vi "Initialize Attributes.vi"(8 "error in (no error)":errorcluster, 10 "Attribute Data":variant, 11 "BNT_DAQmx-MCSV in":refnum<class "BNT_DAQmx-MCSV.lvclass">) -> (0 "error out":errorcluster, 2 "Found?":bool, 3 "BNT_DAQmx-MCSV out":refnum<class "BNT_DAQmx-MCSV.lvclass">)   [LabVIEW 2017, in "BNT_DAQmx.lvlib" / "BNT_DAQmx-MCSV.lvclass"]
doc: "Initialize object attribute.\n\nUnique resources should be allocated elsewhere!"
uses:
  BNT_DAQmx-MCSV.lvclass
  CSPP_Core/Actors/CS++BaseActor/CS++BaseActor.lvclass
  CSPP_Core/Classes/CS++ProcessVariables/ProcessVariable/PV.lvclass
  CSPP_Core/Classes/CS++ProcessVariables/CS++ProcessVariables.lvlib
  CSPP_Core/Actors/CS++DeviceActor/CS++DeviceActor.lvclass
  CSPP_Core/Classes/CS++BaseClasses/Base/CS++Base.lvclass
  CSPP_Core/Classes/CS++BaseClasses/Factory/CS++Factory.lvclass
  CSPP_Core/Libraries/Utilities/CS++Utilities.lvlib
  C:/User/Brand/LVP/TASCA/UTCS/Packages/CSPP_Core/Actors/CS++DeviceActor/CS++DeviceActor.lvclass
  C:/User/Brand/LVP/TASCA/UTCS/Packages/CSPP_Core/Actors/CS++BaseActor/CS++BaseActor.lvclass
  CSPP_Core/Classes/CS++ProcessVariables/PVConnection/PVConnection.lvclass
  C:/User/Brand/LVP/TASCA/UTCS/Packages/CSPP_Core/Classes/CS++BaseClasses/Base/CS++Base.lvclass
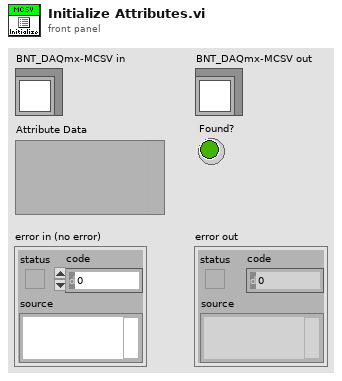
[diagram p1: front panel]
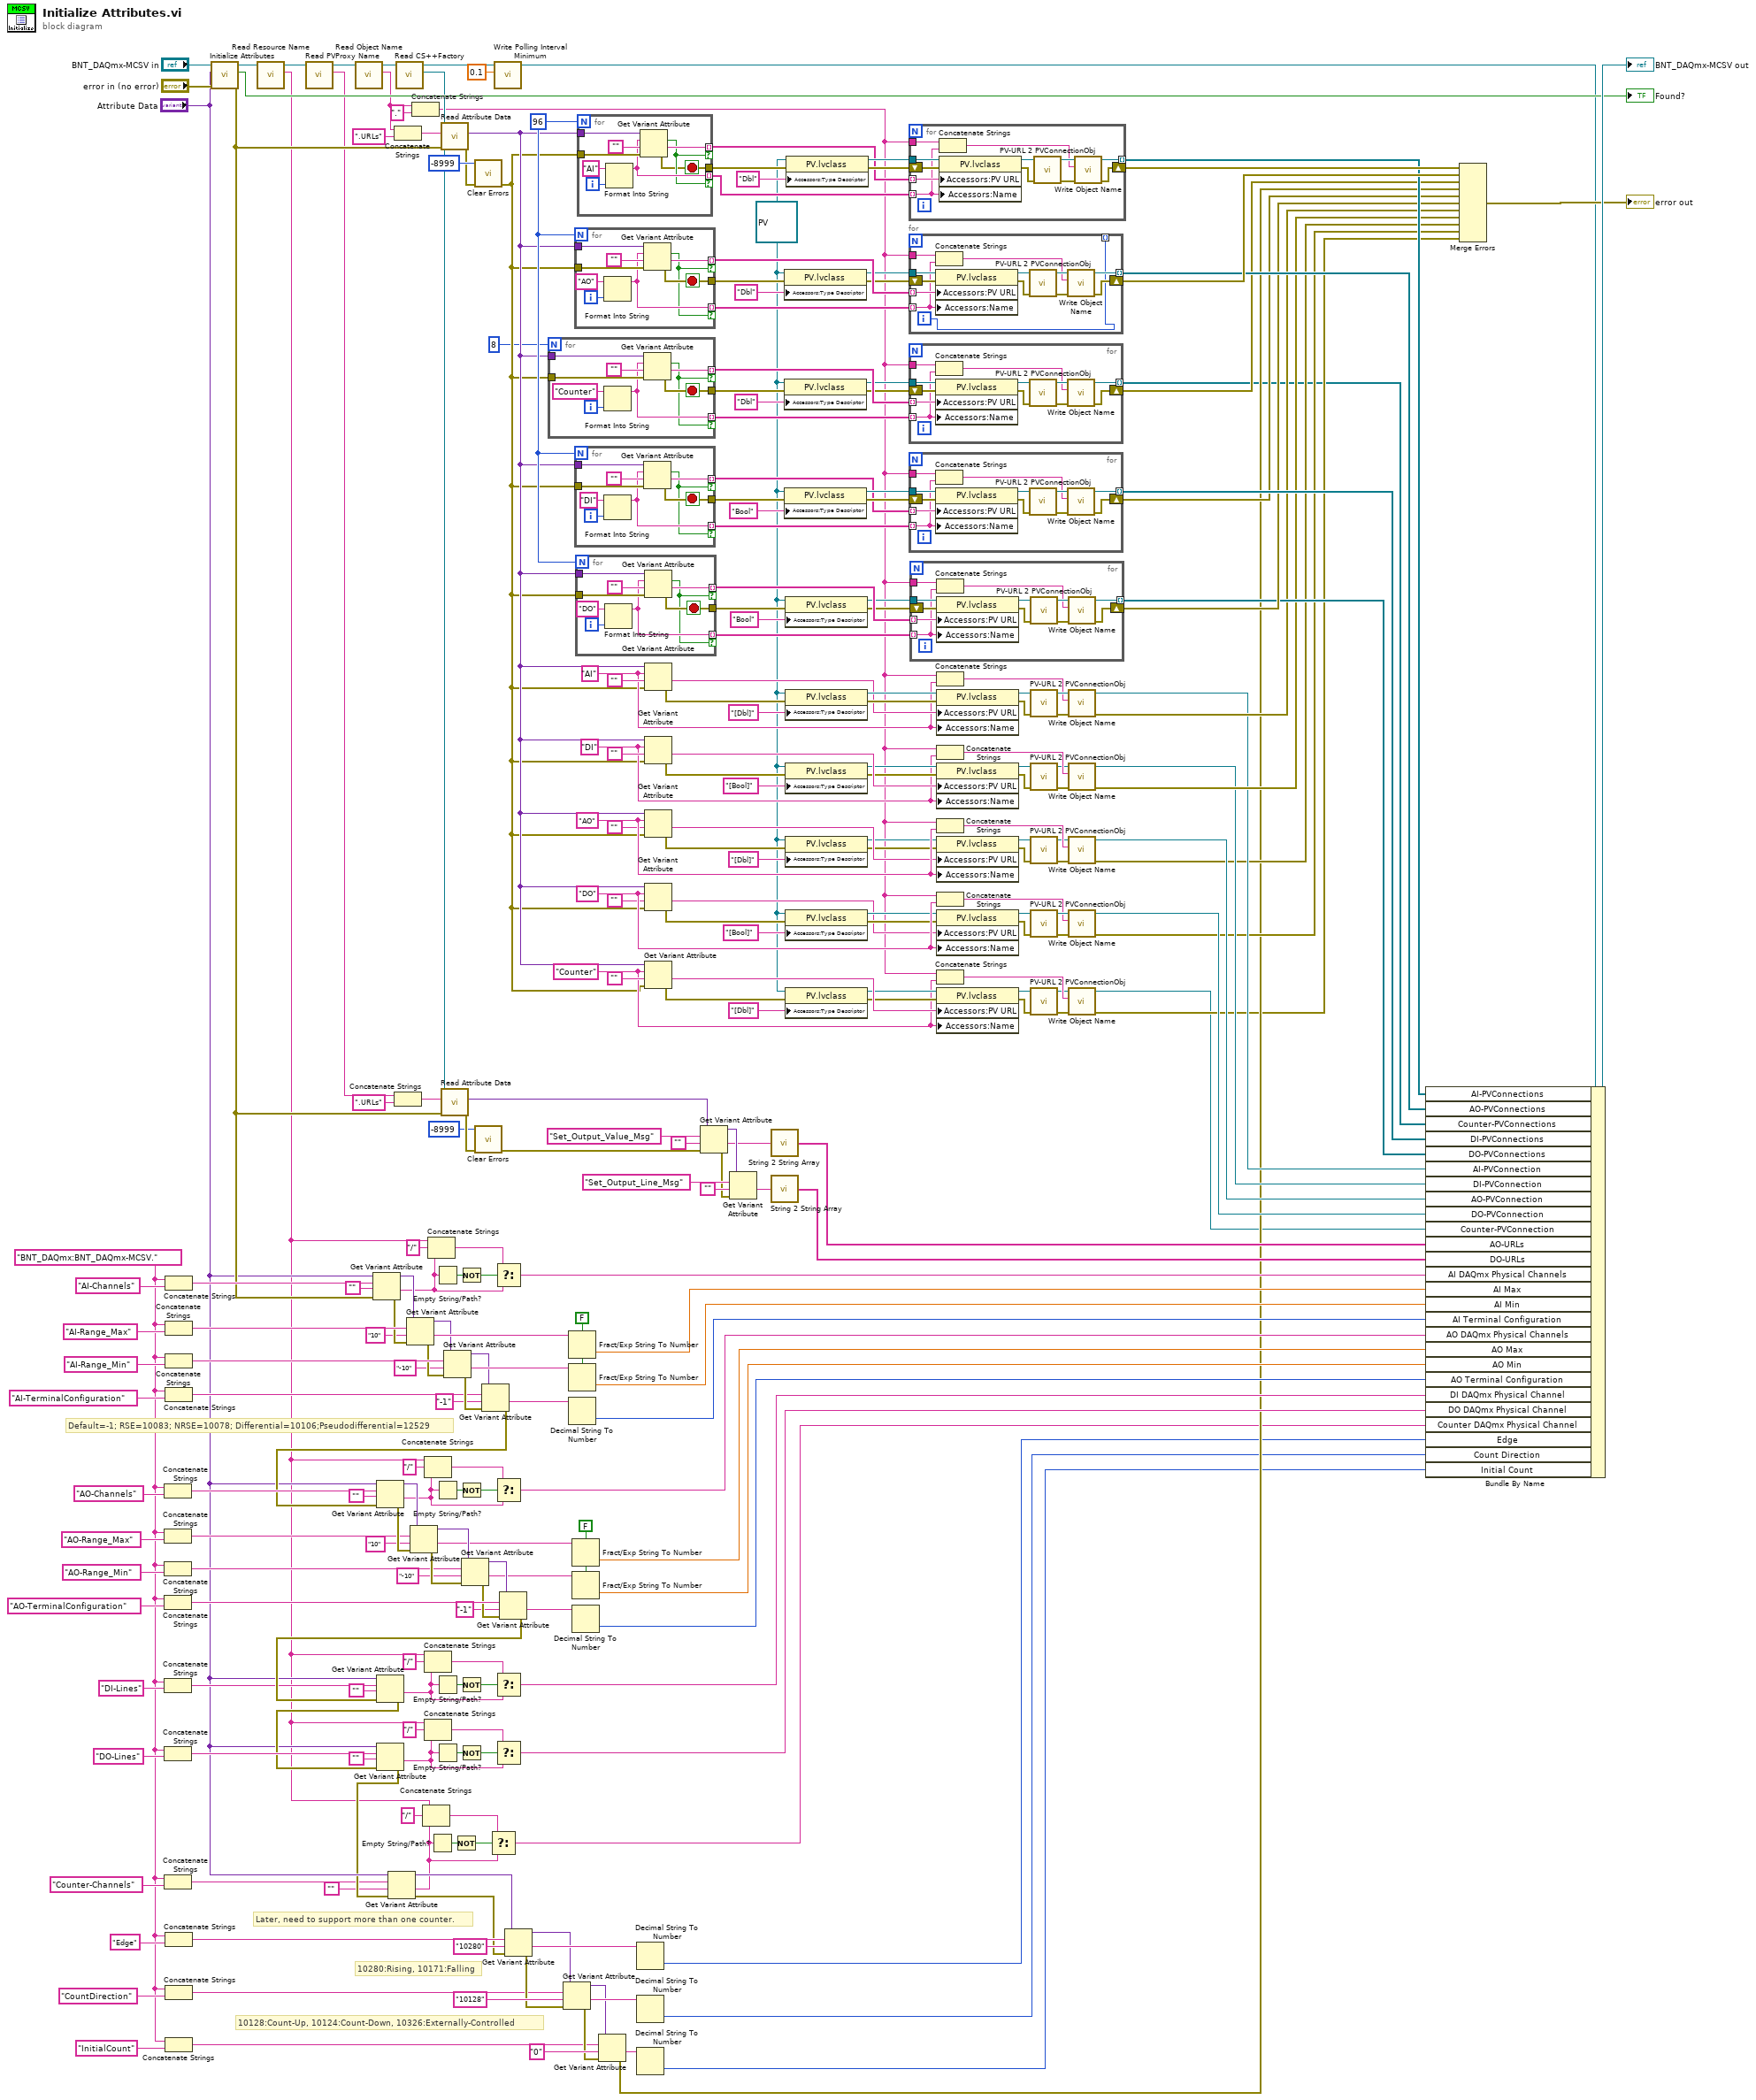
[diagram p0: block diagram]
diagram:
  w16 = "Counter" ("initial string")
  w99 = "DO" ("initial string")
  w100 = "AO" ("initial string")
  w102 = "DI" ("initial string")
  w101 = "AI" ("initial string")
  w221 = FALSE ("use system decimal point (T)")
  w245 = FALSE ("use system decimal point (T)")
  w1 = refnum<class "PV.lvclass"> refnum ("CS++ProcessVariables.lvlib:PV.lvclass")
  w170 = 96
  w40 = "BNT_DAQmx:BNT_DAQmx-MCSV."
  # "Later, need to support more than one counter."
  # "10128:Count-Up, 10124:Count-Down, 10326:Externally-Controlled"
  # "10280:Rising, 10171:Falling"
  # "Default=-1; RSE=10083; NRSE=10078; Differential=10106;Pseudodifferential=12529"
  n1 = Concatenate Strings(w40, "AO-Channels" ("string")) -> (w223:string)
  n2 = Concatenate Strings(w40, "AO-Range_Max" ("string")) -> (w211:string)
  n3 = Concatenate Strings(w40, "AO-Range_Min" ("string")) -> (w214:string)
  n4 = Concatenate Strings(w40, "AO-TerminalConfiguration" ("string")) -> (w219:string)
  n5 = Concatenate Strings(w40, "DI-Lines" ("string")) -> (w152:string)
  n6 = Concatenate Strings(w40, "DO-Lines" ("string")) -> (w157:string)
  n7 = Concatenate Strings(w40, "Counter-Channels" ("string")) -> (w39:string)
  n8 = Concatenate Strings(w40, "AI-Channels" ("string")) -> (w236:string)
  n9 = Concatenate Strings(w40, "AI-Range_Max" ("string")) -> (w266:string)
  n10 = Concatenate Strings(w40, "AI-Range_Min" ("string")) -> (w263:string)
  n11 = Concatenate Strings(w40, "AI-TerminalConfiguration" ("string")) -> (w258:string)
  n12 = Concatenate Strings(w40, "Edge" ("string")) -> (w55:string)
  n13 = Concatenate Strings(w40, "CountDirection" ("string")) -> (w50:string)
  n14 = Concatenate Strings(w40, "InitialCount" ("string")) -> (w52:string)
  n15 = call-parent "Initialize Attributes.vi"("error in (no error)"="error in (no error)", "Attribute Data"="Attribute Data", "CS++DeviceActor in"="BNT_DAQmx-MCSV in") -> ("error out"=w143:errorcluster, "Found?"=→"Found?":bool, "CS++DeviceActor out"=w232:refnum<class "BNT_DAQmx-MCSV.lvclass">)  [unwired: 6 in]
  n16 = call "Read Resource Name.vi"("CS++DeviceActor in"=w232) -> ("Resource Name"=w33:string, "CS++DeviceActor out"=w149:refnum<class "BNT_DAQmx-MCSV.lvclass">)  [unwired: 8 in, 1 out]
  n17 = call "Read PVProxy Name.vi"("CS++BaseActor in"=w149) -> ("PVProxy Name"=w142:string, "CS++BaseActor out"=w148:refnum<class "BNT_DAQmx-MCSV.lvclass">)  [unwired: 8 in, 1 out]
  n18 = call "Read Object Name.vi"("CS++BaseActor in"=w148) -> ("Object Name"=w193:string, "CS++BaseActor out"=w254:refnum<class "BNT_DAQmx-MCSV.lvclass">)  [unwired: 8 in, 1 out]
  n19 = Get Variant Attribute(Variant="Attribute Data", name=w236, default value (empty Variant)="", error in=w143) -> (duplicate Variant=w235:variant, value=w205:string, error out=w234:errorcluster)  [unwired: 1 out]
  n20 = Concatenate Strings(w193, ".URLs" ("string")) -> (w252:string)
  n21 = Concatenate Strings(w142, ".URLs" ("string")) -> (w145:string)
  n22 = call "Read CS++Factory.vi"("CS++BaseActor in"=w254) -> ("CS++Factory"=w141:refnum<class "CS++Factory.lvclass">, "CS++BaseActor out"=w189:refnum<class "BNT_DAQmx-MCSV.lvclass">)  [unwired: 8 in, 1 out]
  n23 = Get Variant Attribute(Variant=w235, name=w266, default value (empty Variant)="10" ("string"), error in=w234) -> (duplicate Variant=w264:variant, value=w265:string, error out=w262:errorcluster)  [unwired: 1 out]
  n24 = Concatenate Strings(w193, "." ("string")) -> (w7:string)
  n25 = Concatenate Strings(w33, "/" ("string"), w205) -> (w203:string)
  n26 = Empty String/Path?(string/path=w205) -> (empty?=w206:bool)
  n27 = call-dynamic "Read Attribute Data.vi"("error in (no error)"=w143, "Object Name"=w252, "CS++Factory in"=w141) -> ("error out"=w190:errorcluster, "Attribute Data"=w6:variant)  [unwired: 6 in, 1 out]
  n28 = call-dynamic "Read Attribute Data.vi"("error in (no error)"=w143, "Object Name"=w145, "CS++Factory in"=w141) -> ("error out"=w147:errorcluster, "Attribute Data"=w139:variant)  [unwired: 6 in, 1 out]
  n29 = Get Variant Attribute(Variant=w264, name=w263, default value (empty Variant)="-10" ("string"), error in=w262) -> (duplicate Variant=w259:variant, value=w261:string, error out=w260:errorcluster)  [unwired: 1 out]
  n30 = Not(x=w206) -> (.not. x?=w204:bool)
  n31 = call <vilib>:"Clear Errors.vi"("error in (no error)"=w190, "specific error code to clear (0: all)"=-8999) -> ("error out"=w5:errorcluster)  [unwired: 4 in, 1 out]
  n32 = call <vilib>:"Clear Errors.vi"("error in (no error)"=w147, "specific error code to clear (0: all)"=-8999) -> ("error out"=w138:errorcluster)  [unwired: 4 in, 1 out]
  n33 = Get Variant Attribute(Variant=w259, name=w258, default value (empty Variant)="-1" ("string"), error in=w260) -> (value=w257:string, error out=w194:errorcluster)  [unwired: 2 out]
  n34 = Get Variant Attribute(Variant="Attribute Data", name=w223, default value (empty Variant)="", error in=w194) -> (duplicate Variant=w224:variant, value=w199:string, error out=w225:errorcluster)  [unwired: 1 out]
  n35 = Get Variant Attribute(Variant=w224, name=w211, default value (empty Variant)="10" ("string"), error in=w225) -> (duplicate Variant=w213:variant, value=w212:string, error out=w215:errorcluster)  [unwired: 1 out]
  n36 = Concatenate Strings(w33, "/" ("string"), w199) -> (w198:string)
  n37 = Empty String/Path?(string/path=w199) -> (empty?=w200:bool)
  n38 = Not(x=w200) -> (.not. x?=w201:bool)
  n39 = Get Variant Attribute(Variant=w213, name=w214, default value (empty Variant)="-10" ("string"), error in=w215) -> (duplicate Variant=w218:variant, value=w216:string, error out=w217:errorcluster)  [unwired: 1 out]
  n40 = call "Write Polling Interval Minimum.vi"("Polling Interval Minimum"=dbl[unit] 0.1, "CS++BaseActor in"=w189) -> ("CS++BaseActor out"=w188:refnum<class "BNT_DAQmx-MCSV.lvclass">)  [unwired: 8 in, 1 out]
  n41 = Select(t=w203, s=w204, f=w205) -> (s? t:f=w202:string)
  n42 = Select(t=w198, s=w201, f=w199) -> (s? t:f=w197:string)
  n43 = Get Variant Attribute(Variant=w218, name=w219, default value (empty Variant)="-1" ("string"), error in=w217) -> (value=w220:string, error out=w163:errorcluster)  [unwired: 2 out]
  n44 = Get Variant Attribute(Variant="Attribute Data", name=w152, default value (empty Variant)="", error in=w163) -> (value=w168:string, error out=w151:errorcluster)  [unwired: 2 out]
  n45 = Get Variant Attribute(Variant="Attribute Data", name=w157, default value (empty Variant)="", error in=w151) -> (value=w154:string, error out=w44:errorcluster)  [unwired: 2 out]
  n46 = Get Variant Attribute(Variant="Attribute Data", name=w39, default value (empty Variant)="", error in=w44) -> (duplicate Variant=w41:variant, value=w32:string, error out=w45:errorcluster)  [unwired: 1 out]
  n47 = Concatenate Strings(w33, "/" ("string"), w32) -> (w37:string)
  n48 = Concatenate Strings(w33, "/" ("string"), w168) -> (w169:string)
  n49 = Concatenate Strings(w33, "/" ("string"), w154) -> (w153:string)
  n50 = Empty String/Path?(string/path=w32) -> (empty?=w35:bool)
  n51 = Empty String/Path?(string/path=w168) -> (empty?=w167:bool)
  n52 = Empty String/Path?(string/path=w154) -> (empty?=w155:bool)
  n53 = Not(x=w35) -> (.not. x?=w36:bool)
  n54 = Not(x=w167) -> (.not. x?=w166:bool)
  n55 = Not(x=w155) -> (.not. x?=w156:bool)
  n56 = Select(t=w37, s=w36, f=w32) -> (s? t:f=w31:string)
  n57 = Select(t=w169, s=w166, f=w168) -> (s? t:f=w162:string)
  n58 = Select(t=w153, s=w156, f=w154) -> (s? t:f=w150:string)
  n59 = Get Variant Attribute(Variant=w41, name=w55, default value (empty Variant)="10280", error in=w45) -> (duplicate Variant=w42:variant, value=w57:string, error out=w56:errorcluster)  [unwired: 1 out]
  n60 = for {
    N: 8 -> [_]
    tunnel: w6 -> [w279]
    tunnel: [w278] -> w12 mode=indexing if=w272
    tunnel: w5 -> [w277]
    tunnel: [w273] -> w11
    tunnel: [w274] -> w13 mode=indexing if=w272
    i -> [w276]
    stop <- w273 stop-if-true
    n61 = Format Into String(initial string="Counter", w276) -> (resulting string=w274:string)  [unwired: 2 in, 1 out]
    n62 = Get Variant Attribute(Variant=w279, name=w274, default value (empty Variant)="", error in=w277) -> (found=w272:bool, value=w278:string, error out=w273:errorcluster)  [unwired: 1 out]
  }
  n63 = Get Variant Attribute(Variant=w42, name=w50, default value (empty Variant)="10128", error in=w56) -> (duplicate Variant=w51:variant, value=w60:string, error out=w53:errorcluster)  [unwired: 1 out]
  n64 = Fract/Exp String To Number(use system decimal point (T)=w245, string=w265) -> (number=w72:dbl)  [unwired: 2 in, 1 out]
  n65 = Fract/Exp String To Number(use system decimal point (T)=w245, string=w261) -> (number=w71:dbl)  [unwired: 2 in, 1 out]
  n66 = Decimal String To Number(string=w257) -> (number=w255:i32)  [unwired: 2 in, 1 out]
  n67 = Fract/Exp String To Number(use system decimal point (T)=w221, string=w212) -> (number=w70:dbl)  [unwired: 2 in, 1 out]
  n68 = Fract/Exp String To Number(use system decimal point (T)=w221, string=w216) -> (number=w69:dbl)  [unwired: 2 in, 1 out]
  n69 = Decimal String To Number(string=w220) -> (number=w207:i32)  [unwired: 2 in, 1 out]
  n70 = for {
    N: w170 -> [_]
    tunnel: w6 -> [w288]
    tunnel: [w287] -> w242 mode=indexing if=w281
    tunnel: w5 -> [w286]
    tunnel: [w282] -> w241
    tunnel: [w283] -> w243 mode=indexing if=w281
    i -> [w285]
    stop <- w282 stop-if-true
    n71 = Format Into String(initial string="AO", w285) -> (resulting string=w283:string)  [unwired: 2 in, 1 out]
    n72 = Get Variant Attribute(Variant=w288, name=w283, default value (empty Variant)="", error in=w286) -> (found=w281:bool, value=w287:string, error out=w282:errorcluster)  [unwired: 1 out]
  }
  n73 = for {
    N: w170 -> [_]
    tunnel: w6 -> [w297]
    tunnel: [w296] -> w182 mode=indexing if=w290
    tunnel: w5 -> [w295]
    tunnel: [w291] -> w183
    tunnel: [w292] -> w181 mode=indexing if=w290
    i -> [w294]
    stop <- w291 stop-if-true
    n74 = Format Into String(initial string="DI", w294) -> (resulting string=w292:string)  [unwired: 2 in, 1 out]
    n75 = Get Variant Attribute(Variant=w297, name=w292, default value (empty Variant)="", error in=w295) -> (found=w290:bool, value=w296:string, error out=w291:errorcluster)  [unwired: 1 out]
  }
  n76 = for {
    N: w170 -> [_]
    tunnel: w6 -> [w306]
    tunnel: [w305] -> w177 mode=indexing if=w299
    tunnel: w5 -> [w304]
    tunnel: [w300] -> w176
    tunnel: [w301] -> w178 mode=indexing if=w299
    i -> [w303]
    stop <- w300 stop-if-true
    n77 = Format Into String(initial string="DO", w303) -> (resulting string=w301:string)  [unwired: 2 in, 1 out]
    n78 = Get Variant Attribute(Variant=w306, name=w301, default value (empty Variant)="", error in=w304) -> (found=w299:bool, value=w305:string, error out=w300:errorcluster)  [unwired: 1 out]
  }
  n79 = for {
    N: w170 -> [_]
    tunnel: w6 -> [w315]
    tunnel: [w314] -> w246 mode=indexing if=w309
    tunnel: w5 -> [w313]
    tunnel: [w308] -> w247
    tunnel: [w310] -> w244 mode=indexing if=w309
    i -> [w312]
    stop <- w308 stop-if-true
    n80 = Format Into String(initial string="AI", w312) -> (resulting string=w310:string)  [unwired: 2 in, 1 out]
    n81 = Get Variant Attribute(Variant=w315, name=w310, default value (empty Variant)="", error in=w313) -> (found=w309:bool, value=w314:string, error out=w308:errorcluster)  [unwired: 1 out]
  }
  n82 = Get Variant Attribute(Variant=w51, name=w52, default value (empty Variant)="0", error in=w53) -> (value=w61:string, error out=w43:errorcluster)  [unwired: 2 out]
  n83 = Decimal String To Number(string=w57) -> (number=w30:i32)  [unwired: 2 in, 1 out]
  n84 = Decimal String To Number(string=w60) -> (number=w29:i32)  [unwired: 2 in, 1 out]
  n85 = Decimal String To Number(string=w61) -> (number=w28:i32)  [unwired: 2 in, 1 out]
  n86 = Get Variant Attribute(Variant=w6, name=w101, default value (empty Variant)="", error in=w5) -> (value=w124:string, error out=w125:errorcluster)  [unwired: 2 out]
  n87 = Get Variant Attribute(Variant=w6, name=w102, default value (empty Variant)="", error in=w5) -> (value=w110:string, error out=w109:errorcluster)  [unwired: 2 out]
  n88 = Get Variant Attribute(Variant=w6, name=w100, default value (empty Variant)="", error in=w5) -> (value=w81:string, error out=w80:errorcluster)  [unwired: 2 out]
  n89 = Get Variant Attribute(Variant=w6, name=w99, default value (empty Variant)="", error in=w5) -> (value=w94:string, error out=w95:errorcluster)  [unwired: 2 out]
  n90 = Get Variant Attribute(Variant=w6, name=w16, default value (empty Variant)="", error in=w5) -> (value=w21:string, error out=w20:errorcluster)  [unwired: 2 out]
  n91 = Get Variant Attribute(Variant=w139, name="Set_Output_Value_Msg", default value (empty Variant)="", error in=w138) -> (duplicate Variant=w134:variant, value=w132:string, error out=w133:errorcluster)  [unwired: 1 out]
  n92 = Get Variant Attribute(Variant=w134, name="Set_Output_Line_Msg", default value (empty Variant)="", error in=w133) -> (value=w131:string)  [unwired: 3 out]
  n93 = call "String 2 String Array.vi"("String"=w132) -> ("Substrings"=w130:string[])  [unwired: 1 in]
  n94 = call "String 2 String Array.vi"("String"=w131) -> ("Substrings"=w129:string[])  [unwired: 1 in]
  n95 = property class="PV.lvclass"(reference=w1, error in=w241, "Accessors:Type Descriptor"="Dbl" ("Type Descriptor")) -> (reference out=w239:refnum<class "PV.lvclass">, error out=w240:errorcluster)
  n96 = property class="PV.lvclass"(reference=w1, error in=w11, "Accessors:Type Descriptor"="Dbl" ("Type Descriptor")) -> (reference out=w9:refnum<class "PV.lvclass">, error out=w10:errorcluster)
  n97 = property class="PV.lvclass"(reference=w1, error in=w183, "Accessors:Type Descriptor"="Bool" ("Type Descriptor")) -> (reference out=w185:refnum<class "PV.lvclass">, error out=w184:errorcluster)
  n98 = property class="PV.lvclass"(reference=w1, error in=w176, "Accessors:Type Descriptor"="Bool" ("Type Descriptor")) -> (reference out=w174:refnum<class "PV.lvclass">, error out=w175:errorcluster)
  n99 = property class="PV.lvclass"(reference=w1, error in=w125, "Accessors:Type Descriptor"="[Dbl]" ("Type Descriptor")) -> (reference out=w127:refnum<class "PV.lvclass">, error out=w126:errorcluster)
  n100 = property class="PV.lvclass"(reference=w1, error in=w109, "Accessors:Type Descriptor"="[Bool]" ("Type Descriptor")) -> (reference out=w107:refnum<class "PV.lvclass">, error out=w108:errorcluster)
  n101 = property class="PV.lvclass"(reference=w1, error in=w80, "Accessors:Type Descriptor"="[Dbl]" ("Type Descriptor")) -> (reference out=w78:refnum<class "PV.lvclass">, error out=w79:errorcluster)
  n102 = property class="PV.lvclass"(reference=w1, error in=w95, "Accessors:Type Descriptor"="[Bool]" ("Type Descriptor")) -> (reference out=w97:refnum<class "PV.lvclass">, error out=w96:errorcluster)
  n103 = property class="PV.lvclass"(reference=w1, error in=w20, "Accessors:Type Descriptor"="[Dbl]" ("Type Descriptor")) -> (reference out=w18:refnum<class "PV.lvclass">, error out=w19:errorcluster)
  n104 = property class="PV.lvclass"(reference=w1, error in=w247, "Accessors:Type Descriptor"="Dbl" ("Type Descriptor")) -> (reference out=w249:refnum<class "PV.lvclass">, error out=w248:errorcluster)
  n105 = for {
    tunnel: w249 -> [w327]
    tunnel: w246 -> [w326] mode=indexing
    tunnel: [w320] -> w196 mode=indexing
    shift-right: [w318] -> w229
    shift-left: w248 -> [w324]
    tunnel: w244 -> [w322] mode=indexing
    tunnel: w7 -> [w323]
    n106 = Concatenate Strings(w323, w322) -> (w317:string)
    n107 = property class="PV.lvclass"(reference=w327, error in=w324, "Accessors:PV URL"=w326, "Accessors:Name"=w322) -> (reference out=w328:refnum<class "PV.lvclass">, error out=w325:errorcluster)
    n108 = call "PV-URL 2 PVConnectionObj.vi"("Error In"=w325, "PV"=w328) -> ("Error Out"=w319:errorcluster, "PVConnection"=w321:refnum<class "PVConnection.lvclass">)  [unwired: 7 in, 1 out]
    n109 = call "Write Object Name.vi"("error in (no error)"=w319, "Object Name"=w317, "Base in"=w321) -> ("error out"=w318:errorcluster, "Base out"=w320:refnum<class "PVConnection.lvclass">)  [unwired: 7 in]
  }
  n110 = for {
    tunnel: w239 -> [w340]
    tunnel: w242 -> [w339] mode=indexing
    tunnel: [w331] -> w195 mode=indexing
    shift-right: [w330] -> w230
    shift-left: w240 -> [w337]
    tunnel: w243 -> [w336] mode=indexing
    tunnel: w7 -> [w335]
    tunnel: [w329] -> _ mode=indexing
    i -> [w329]
    n111 = Concatenate Strings(w335, w336) -> (w332:string)
    n112 = property class="PV.lvclass"(reference=w340, error in=w337, "Accessors:PV URL"=w339, "Accessors:Name"=w336) -> (reference out=w341:refnum<class "PV.lvclass">, error out=w338:errorcluster)
    n113 = call "PV-URL 2 PVConnectionObj.vi"("Error In"=w338, "PV"=w341) -> ("Error Out"=w334:errorcluster, "PVConnection"=w333:refnum<class "PVConnection.lvclass">)  [unwired: 7 in, 1 out]
    n114 = call "Write Object Name.vi"("error in (no error)"=w334, "Object Name"=w332, "Base in"=w333) -> ("error out"=w330:errorcluster, "Base out"=w331:refnum<class "PVConnection.lvclass">)  [unwired: 7 in]
  }
  n115 = for {
    tunnel: w9 -> [w352]
    tunnel: w12 -> [w351] mode=indexing
    tunnel: [w343] -> w2 mode=indexing
    shift-right: [w342] -> w3
    shift-left: w10 -> [w349]
    tunnel: w13 -> [w348] mode=indexing
    tunnel: w7 -> [w347]
    n116 = Concatenate Strings(w347, w348) -> (w344:string)
    n117 = property class="PV.lvclass"(reference=w352, error in=w349, "Accessors:PV URL"=w351, "Accessors:Name"=w348) -> (reference out=w353:refnum<class "PV.lvclass">, error out=w350:errorcluster)
    n118 = call "PV-URL 2 PVConnectionObj.vi"("Error In"=w350, "PV"=w353) -> ("Error Out"=w346:errorcluster, "PVConnection"=w345:refnum<class "PVConnection.lvclass">)  [unwired: 7 in, 1 out]
    n119 = call "Write Object Name.vi"("error in (no error)"=w346, "Object Name"=w344, "Base in"=w345) -> ("error out"=w342:errorcluster, "Base out"=w343:refnum<class "PVConnection.lvclass">)  [unwired: 7 in]
  }
  n120 = for {
    tunnel: w185 -> [w364]
    tunnel: w182 -> [w363] mode=indexing
    tunnel: [w355] -> w180 mode=indexing
    shift-right: [w354] -> w179
    shift-left: w184 -> [w361]
    tunnel: w181 -> [w360] mode=indexing
    tunnel: w7 -> [w359]
    n121 = Concatenate Strings(w359, w360) -> (w356:string)
    n122 = property class="PV.lvclass"(reference=w364, error in=w361, "Accessors:PV URL"=w363, "Accessors:Name"=w360) -> (reference out=w365:refnum<class "PV.lvclass">, error out=w362:errorcluster)
    n123 = call "PV-URL 2 PVConnectionObj.vi"("Error In"=w362, "PV"=w365) -> ("Error Out"=w358:errorcluster, "PVConnection"=w357:refnum<class "PVConnection.lvclass">)  [unwired: 7 in, 1 out]
    n124 = call "Write Object Name.vi"("error in (no error)"=w358, "Object Name"=w356, "Base in"=w357) -> ("error out"=w354:errorcluster, "Base out"=w355:refnum<class "PVConnection.lvclass">)  [unwired: 7 in]
  }
  n125 = for {
    tunnel: w174 -> [w376]
    tunnel: w177 -> [w375] mode=indexing
    tunnel: [w367] -> w171 mode=indexing
    shift-right: [w366] -> w172
    shift-left: w175 -> [w373]
    tunnel: w178 -> [w372] mode=indexing
    tunnel: w7 -> [w371]
    n126 = Concatenate Strings(w371, w372) -> (w368:string)
    n127 = property class="PV.lvclass"(reference=w376, error in=w373, "Accessors:PV URL"=w375, "Accessors:Name"=w372) -> (reference out=w377:refnum<class "PV.lvclass">, error out=w374:errorcluster)
    n128 = call "PV-URL 2 PVConnectionObj.vi"("Error In"=w374, "PV"=w377) -> ("Error Out"=w370:errorcluster, "PVConnection"=w369:refnum<class "PVConnection.lvclass">)  [unwired: 7 in, 1 out]
    n129 = call "Write Object Name.vi"("error in (no error)"=w370, "Object Name"=w368, "Base in"=w369) -> ("error out"=w366:errorcluster, "Base out"=w367:refnum<class "PVConnection.lvclass">)  [unwired: 7 in]
  }
  n130 = Concatenate Strings(w7, w101) -> (w118:string)
  n131 = property class="PV.lvclass"(reference=w127, error in=w126, "Accessors:PV URL"=w124, "Accessors:Name"=w101) -> (reference out=w122:refnum<class "PV.lvclass">, error out=w121:errorcluster)
  n132 = Concatenate Strings(w7, w102) -> (w116:string)
  n133 = property class="PV.lvclass"(reference=w107, error in=w108, "Accessors:PV URL"=w110, "Accessors:Name"=w102) -> (reference out=w112:refnum<class "PV.lvclass">, error out=w113:errorcluster)
  n134 = Concatenate Strings(w7, w100) -> (w87:string)
  n135 = property class="PV.lvclass"(reference=w78, error in=w79, "Accessors:PV URL"=w81, "Accessors:Name"=w100) -> (reference out=w83:refnum<class "PV.lvclass">, error out=w84:errorcluster)
  n136 = Concatenate Strings(w7, w99) -> (w88:string)
  n137 = property class="PV.lvclass"(reference=w97, error in=w96, "Accessors:PV URL"=w94, "Accessors:Name"=w99) -> (reference out=w92:refnum<class "PV.lvclass">, error out=w91:errorcluster)
  n138 = Concatenate Strings(w7, w16) -> (w27:string)
  n139 = property class="PV.lvclass"(reference=w18, error in=w19, "Accessors:PV URL"=w21, "Accessors:Name"=w16) -> (reference out=w23:refnum<class "PV.lvclass">, error out=w24:errorcluster)
  n140 = call "PV-URL 2 PVConnectionObj.vi"("Error In"=w121, "PV"=w122) -> ("Error Out"=w120:errorcluster, "PVConnection"=w119:refnum<class "PVConnection.lvclass">)  [unwired: 7 in, 1 out]
  n141 = call "PV-URL 2 PVConnectionObj.vi"("Error In"=w113, "PV"=w112) -> ("Error Out"=w114:errorcluster, "PVConnection"=w115:refnum<class "PVConnection.lvclass">)  [unwired: 7 in, 1 out]
  n142 = call "PV-URL 2 PVConnectionObj.vi"("Error In"=w84, "PV"=w83) -> ("Error Out"=w85:errorcluster, "PVConnection"=w86:refnum<class "PVConnection.lvclass">)  [unwired: 7 in, 1 out]
  n143 = call "PV-URL 2 PVConnectionObj.vi"("Error In"=w91, "PV"=w92) -> ("Error Out"=w90:errorcluster, "PVConnection"=w89:refnum<class "PVConnection.lvclass">)  [unwired: 7 in, 1 out]
  n144 = call "PV-URL 2 PVConnectionObj.vi"("Error In"=w24, "PV"=w23) -> ("Error Out"=w25:errorcluster, "PVConnection"=w26:refnum<class "PVConnection.lvclass">)  [unwired: 7 in, 1 out]
  n145 = call "Write Object Name.vi"("error in (no error)"=w120, "Object Name"=w118, "Base in"=w119) -> ("error out"=w117:errorcluster, "Base out"=w104:refnum<class "PVConnection.lvclass">)  [unwired: 7 in]
  n146 = call "Write Object Name.vi"("error in (no error)"=w114, "Object Name"=w116, "Base in"=w115) -> ("error out"=w105:errorcluster, "Base out"=w103:refnum<class "PVConnection.lvclass">)  [unwired: 7 in]
  n147 = call "Write Object Name.vi"("error in (no error)"=w85, "Object Name"=w87, "Base in"=w86) -> ("error out"=w74:errorcluster, "Base out"=w76:refnum<class "PVConnection.lvclass">)  [unwired: 7 in]
  n148 = call "Write Object Name.vi"("error in (no error)"=w90, "Object Name"=w88, "Base in"=w89) -> ("error out"=w73:errorcluster, "Base out"=w75:refnum<class "PVConnection.lvclass">)  [unwired: 7 in]
  n149 = call "Write Object Name.vi"("error in (no error)"=w25, "Object Name"=w27, "Base in"=w26) -> ("error out"=w15:errorcluster, "Base out"=w14:refnum<class "PVConnection.lvclass">)  [unwired: 7 in]
  n150 = Bundle By Name(cluster=w188, "AI-PVConnections"=w196, "AO-PVConnections"=w195, "Counter-PVConnections"=w2, "DI-PVConnections"=w180, "DO-PVConnections"=w171, "AI-PVConnection"=w104, "DI-PVConnection"=w103, "AO-PVConnection"=w76, "DO-PVConnection"=w75, "Counter-PVConnection"=w14, "AO-URLs"=w130, "DO-URLs"=w129, "AI DAQmx Physical Channels"=w202, "AI Max"=w72, "AI Min"=w71, "AI Terminal Configuration"=w255, "AO DAQmx Physical Channels"=w197, "AO Max"=w70, "AO Min"=w69, "AO Terminal Configuration"=w207, "DI DAQmx Physical Channel"=w162, "DO DAQmx Physical Channel"=w150, "Counter DAQmx Physical Channel"=w31, "Edge"=w30, "Count Direction"=w29, "Initial Count"=w28) -> (→"BNT_DAQmx-MCSV out":refnum<class "BNT_DAQmx-MCSV.lvclass">)
  n151 = Merge Errors(w229, w230, w3, w43, w179, w172, w117, w105, w74, w73, w15) -> (→"error out":errorcluster)
